vi "Read Key File.vi"(7 "Key Type":T1, 8 "Error In":errorcluster, 11 "Key File":path) -> (0 "Error Out":errorcluster, 3 "Key Data":string)   [LabVIEW 2017, in "Tests.lvlib"]
uses:
  Tests.lvlib
  SSH Key Types.ctl
  <vilib>/Utility/sysdir.llb/System Directory Type.ctl
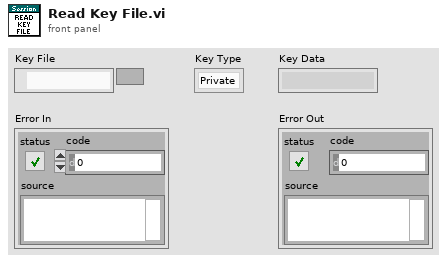
[diagram p1: front panel]
types:
  T1 = typedef "Tests.lvlib/SSH Key Types.ctl" = enum16{"Private", "Public"}
  T2 = enum16{"open", "replace", "create", "open or create", "replace or create", "replace or create with confirmation"}
  T3 = typedef "System Directory Type.ctl" = i32
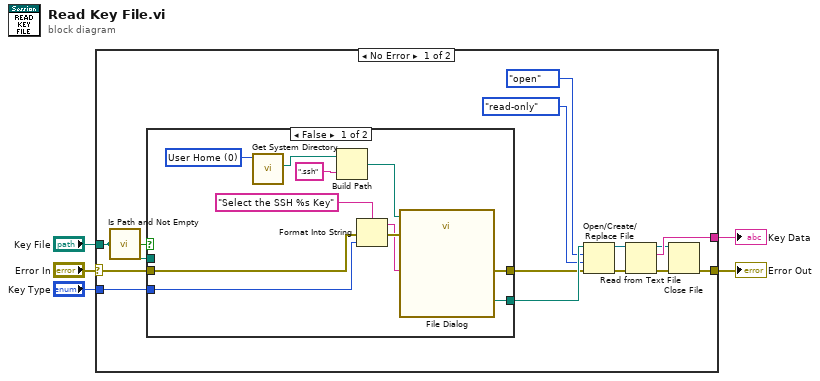
[diagram p0: block diagram]
diagram:
  n1 = case shown="No Error" "Error In" {
    selector: "Error In" -> [w7 w33]
    tunnel: [w19 w33] -> w5
    tunnel: "Key File" -> [w18 _]
    tunnel: [w14 _] -> w3
    tunnel: "Key Type" -> [w6 _]
    frame No Error {
      n2 = call <vilib>:"Is Path and Not Empty.vi"("path"=w18) -> ("Is Path and Not Empty?"=w17:bool)  [unwired: 4 in]
      n3 = case shown="False" w17 {
        tunnel: w7 -> [w30 w31]
        tunnel: [w29 w31] -> w15
        tunnel: [w28 w32] -> w16
        tunnel: w18 -> [_ w32]
        tunnel: w6 -> [w22 _]
        frame False {
          w27 = T3 0 items=["User Home"=0, "User Desktop"=1, "User Documents"=2, "User Application Data"=3, "User Preferences"=4, "User Temporary"=5, "Public Documents"=6, "Public Application Data"=7, "Public Preferences"=8, "Public Cache"=13, "System Core Libraries"=9, "System Installed Libraries"=10, "Application Files"=11, "Boot Volume Root"=12] ("system directory type")
          n4 = call <vilib>:"Get System Directory.vi"("system directory type"=w27) -> ("system directory"=w26:path)  [unwired: 10 in]
          n5 = Build Path(base path=w26, name or relative path=".ssh") -> (appended path=w24:path)
          n6 = Format Into String(format string="Select the SSH %s Key", error in=w30, w22) -> (resulting string=w20:string, error out=w23:errorcluster)  [unwired: 1 in]
          n7 = call "File Dialog"("start path"=w24, "prompt"=w20, "error in"=w23) -> ("selected path"=w28:path, "error out"=w29:errorcluster)  [unwired: 9 in, 2 out]
        }
        frame True {
        }
      }
      n8 = Open/Create/Replace File(file path (use dialog)=w16, error in=w15, operation (0:open)=T2."open", access (0:read/write)=enum16{"read/write", "read-only", "write-only"}."read-only") -> (refnum out=w10:refnum<file>, error out=w11:errorcluster)  [unwired: 2 in, 1 out]
      n9 = Read from Text File(file (use dialog)=w10, error in=w11) -> (refnum out=w13:refnum<file>, text=w14:string, error out=w12:errorcluster)  [unwired: 2 in, 1 out]
      n10 = Close File(refnum=w13, error in=w12) -> (error out=w19:errorcluster)  [unwired: 1 out]
    }
    frame Error {
    }
  }
  "Error Out" <- w5
  "Key Data" <- w3
